vi "p1.vi"() -> ()   [LabVIEW 2025, in "d7.lvlib"]
uses:
  d7.lvlib
  <vilib>/regexp/Match Regular Expression.xnode
  AOC/AOC.lvlib
panel:
  out "Answer":u64=1141028
  in  "Example":string="123 -> x\n456 -> y\nx AND y -> d\nx OR y -> e\nx LSHIFT 2 -> f\ny RSHIFT 2 -> g\nNOT x -> h\nNOT y -> i"
  in  "Example":bool=TRUE
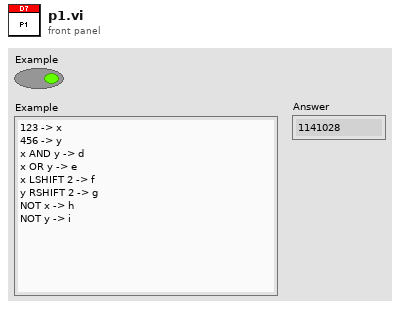
[diagram p1: front panel]
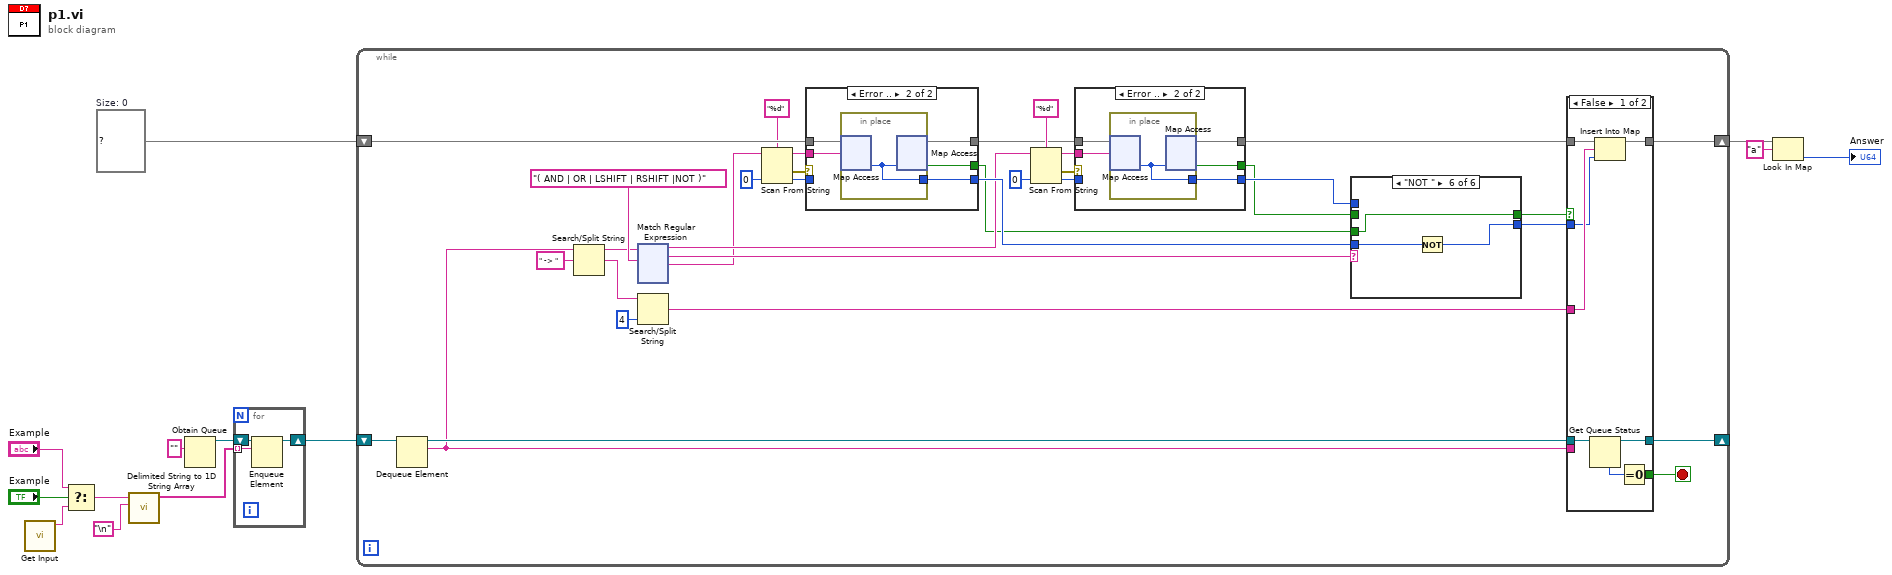
[diagram p0: block diagram]
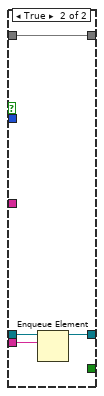
[diagram p2: hidden frame]
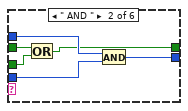
[diagram p4: hidden frame]
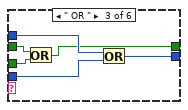
[diagram p5: hidden frame]
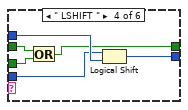
[diagram p6: hidden frame]
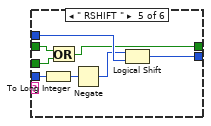
[diagram p7: hidden frame]
diagram:
  w8 = map{string, u16} {}  # Size: 0
  n1 = call "Get Input.vi"() -> ("Input"=w13:string)  [unwired: 11 in]
  n2 = Select(t="Example", s="Example", f=w13) -> (s? t:f=w10:string)
  n3 = call <vilib>:"Delimited String to 1D String Array.vi"("delimiter"="\n", "delimited string"=w10) -> ("string array"=w2:string[])  [unwired: 9 in]
  n4 = Obtain Queue(element data type="" ("s? t:f")) -> (queue out=w3:refnum<queue>)  [unwired: 4 in, 2 out]
  n5 = for {
    tunnel: w2 -> [w16] mode=indexing
    shift-right: [w14] -> w1
    shift-left: w3 -> [w15]
    n6 = Enqueue Element(queue=w15, element=w16) -> (queue out=w14:refnum<queue>)  [unwired: 2 in, 2 out]
  }
  n7 = while {
    shift-right: [w45] -> w7
    shift-left: w8 -> [w42]
    shift-right: [w23] -> _
    shift-left: w1 -> [w25]
    stop <- w22 stop-if-true
    n8 = Dequeue Element(queue=w25) -> (queue out=w24:refnum<queue>, element=w17:string)  [unwired: 2 in, 2 out]
    n9 = Search/Split String(string=w17, search string/char (-)=" -> ") -> (substring before match=w49:string, match + rest of string=w47:string)  [unwired: 1 in, 1 out]
    n10 = xnode "Match Regular Expression"("input string"=w49, "regular expression"="( AND | OR | LSHIFT | RSHIFT |NOT )") -> ("before match"=w27:string, "whole match"=w43:string, "after match"=w26:string)  [unwired: 4 in, 2 out]
    n11 = Search/Split String(string=w47, offset (0)=4) -> (match + rest of string=w44:string)  [unwired: 1 in, 2 out]
    n12 = Scan From String(format string="%d", input string=w26, default 1=u16 0 ("default value 14")) -> (remaining string=w36:string, error out=w38:errorcluster, output 1=w37:u16)  [unwired: 2 in, 1 out]
    n13 = case shown="Error .." w38 {
      tunnel: w42 -> [w103 w108]
      tunnel: [w102 w107] -> w41
      tunnel: [w103 w106] -> w30
      tunnel: w36 -> [_ w105]
      tunnel: w37 -> [w102 _]
      tunnel: [_ w104] -> w20
      frame #0 {
      }
      frame #1 {
        n14 = in-place {
          in-place-border: [w109] -> w107
          n15 = in-place-map #1(w108, w105) -> (w109:u16)  [unwired: 1 in, 1 out]
          n16 = in-place-map #1(w109) -> (w106:map{string, u16}, w104:bool)  [unwired: 1 in, 1 out]
        }
      }
    }
    n17 = Scan From String(format string="%d", input string=w27, default 1=u16 0 ("default value 14")) -> (remaining string=w31:string, error out=w33:errorcluster, output 1=w32:u16)  [unwired: 2 in, 1 out]
    n18 = case shown="Error .." w33 {
      tunnel: w30 -> [w95 w100]
      tunnel: [w94 w99] -> w28
      tunnel: [w95 w98] -> w29
      tunnel: w31 -> [_ w97]
      tunnel: w32 -> [w94 _]
      tunnel: [_ w96] -> w19
      frame #0 {
      }
      frame #1 {
        n19 = in-place {
          in-place-border: [w101] -> w99
          n20 = in-place-map #2(w100, w97) -> (w101:u16)  [unwired: 1 in, 1 out]
          n21 = in-place-map #2(w101) -> (w98:map{string, u16}, w96:bool)  [unwired: 1 in, 1 out]
        }
      }
    }
    n22 = case shown="\"NOT \"" w43 {
      tunnel: [w64 w68 w74 w82 w90 w92] -> w21
      tunnel: w41 -> [_ w69 w75 w80 w88 w93]
      tunnel: w28 -> [w64 w70 w76 w81 w89 _]
      tunnel: w20 -> [_ w66 w72 w79 w84 w91]
      tunnel: w19 -> [w63 w67 w73 w78 w85 _]
      tunnel: [w63 w65 w71 w77 w83 w91] -> w18
      frame Default {
      }
      frame " AND " {
        n23 = Or(x=w67, y=w66) -> (x .or. y?=w65:bool)
        n24 = And(x=w70, y=w69) -> (x .and. y?=w68:u16)
      }
      frame " OR " {
        n25 = Or(x=w73, y=w72) -> (x .or. y?=w71:bool)
        n26 = Or(x=w76, y=w75) -> (x .or. y?=w74:u16)
      }
      frame " LSHIFT " {
        n27 = Or(x=w78, y=w79) -> (x .or. y?=w77:bool)
        n28 = Logical Shift(y=w80, x=w81) -> (x << y=w82:u16)
      }
      frame " RSHIFT " {
        n29 = To Long Integer(number=w88) -> (32bit integer=w87:i32)
        n30 = Or(x=w85, y=w84) -> (x .or. y?=w83:bool)
        n31 = Negate(x=w87) -> (-x=w86:i32)
        n32 = Logical Shift(y=w86, x=w89) -> (x << y=w90:u16)
      }
      frame "NOT " {
        n33 = Not(x=w93) -> (.not. x?=w92:u16)
      }
    }
    n34 = case shown="False" w18 {
      tunnel: [w58 w62] -> w45
      tunnel: w44 -> [w57 _]
      tunnel: w29 -> [w56 w62]
      tunnel: w24 -> [w55 w61]
      tunnel: [w54 w60] -> w23
      tunnel: [w53 _] -> w22
      tunnel: w21 -> [w52 _]
      tunnel: w17 -> [_ w59]
      frame False {
        n35 = Get Queue Status(queue=w55) -> (queue out=w54:refnum<queue>, # elements in queue=w51:i32)  [unwired: 2 in, 6 out]
        n36 = Insert Into Map(map in=w56, key=w57, value=w52) -> (map out=w58:map{string, u16})  [unwired: 2 out]
        n37 = Equal To 0?(x=w51) -> (x = 0?=w53:bool)
      }
      frame True {
        n38 = Enqueue Element(queue=w61, element=w59) -> (queue out=w60:refnum<queue>)  [unwired: 2 in, 2 out]
      }
    }
  }
  n39 = Look In Map(map=w7, key="a") -> (value=→"Answer":u16)  [unwired: 1 in, 1 out]
